vi "Motor_Encoder_UART_V1.vi"() -> ()   [LabVIEW 2025]
uses:
  <vilib>/Instr/_visa.llb/VISA Configure Serial Port (Instr).vi
panel:
  in  "VISA resource name":refnum<visa-resource-name>
  out "error out":errorcluster
  in  "write":bool
  in  "buffer size":u32=256
  in  "timeout (ms)":u32=10000
  in  "flow control":u16
  in  "stop bits":u16=10
  in  "parity":u16(ring) items=["None", "Odd", "Even", "Mark", "Space"]
  in  "data bits":u16=8 min=5 max=8 step=1
  in  "baud rate":u32=9600
  out "READ":string
  in  "SET-POINT":string
  in  "stop":bool
  # "Control motor - encoder Arduino UNO"
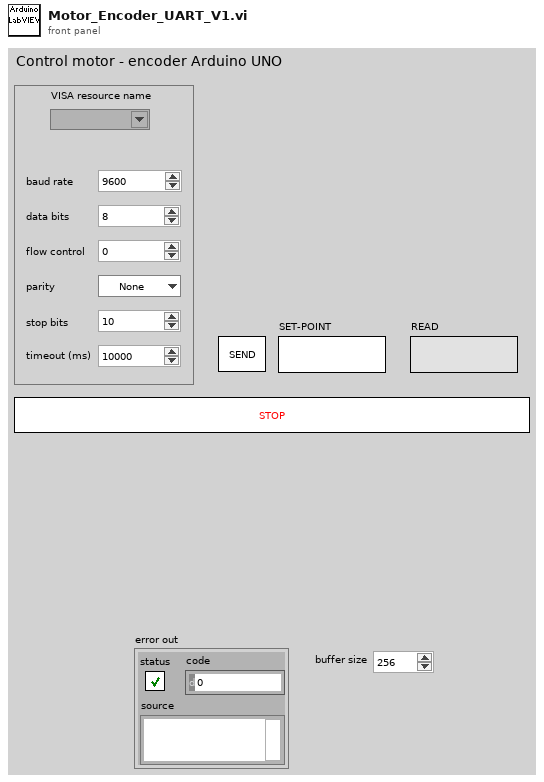
[diagram p1: front panel]
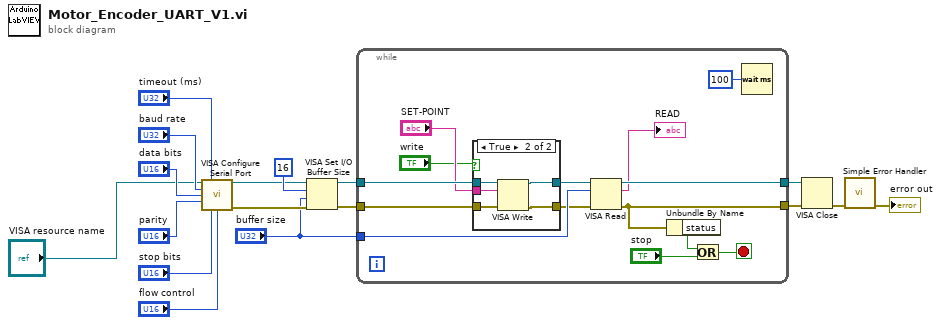
[diagram p0: block diagram]
diagram:
  n1 = call-poly "VISA Configure Serial Port"("VISA resource name"="VISA resource name", "timeout (10sec)"="timeout (ms)", "baud rate (9600)"="baud rate", "data bits (8)"="data bits", "parity (0:none)"="parity", "stop bits (10: 1 bit)"="stop bits", "flow control (0:none)"="flow control") -> ("VISA resource name out"=w8:refnum<visa-resource-name>, "error out"=w7:errorcluster)  [unwired: 7 in]
  n2 = VISA Set I/O Buffer Size(VISA resource name=w8, mask (16)=u16 16 ("I/O Receive\nBuffer mask"), size (4096)="buffer size", error in (no error)=w7) -> (VISA resource name out=w6:refnum<visa-resource-name>, error out=w5:errorcluster)
  n3 = while {
    tunnel: w6 -> [w25]
    tunnel: w5 -> [w24]
    tunnel: [w26] -> w17
    tunnel: [w28] -> w16
    tunnel: "buffer size" -> [w27]
    stop <- w29 stop-if-true
    n4 = case shown="True" "write" {
      tunnel: w25 -> [w33 w38]
      tunnel: w24 -> [w32 w37]
      tunnel: [w33 w36] -> w23
      tunnel: [w32 w35] -> w22
      tunnel: "SET-POINT" -> [_ w34]
      frame False {
      }
      frame True {
        n5 = VISA Write(VISA resource name=w38, write buffer=w34, error in (no error)=w37) -> (VISA resource name out=w36:refnum<visa-resource-name>, error out=w35:errorcluster)  [unwired: 1 out]
      }
    }
    n6 = VISA Read(VISA resource name=w23, byte count=w27, error in (no error)=w22) -> (VISA resource name out=w26:refnum<visa-resource-name>, read buffer=→"READ":string, error out=w28:errorcluster)  [unwired: 1 out]
    n7 = Unbundle By Name(w28) -> ("status"=w31:bool)
    n8 = Or(x=w31, y="stop") -> (x .or. y?=w29:bool)
    n9 = Wait (ms)(milliseconds to wait=u32 100) -> ()  [unwired: 1 out]
  }
  n10 = VISA Close(VISA resource name=w17, error in (no error)=w16) -> (error out=w3:errorcluster)
  n11 = call <vilib>:"Simple Error Handler.vi"("error in (no error)"=w3) -> ("error out"=→"error out":errorcluster)  [unwired: 4 in, 4 out]
